vi "Decompose Map - Variant Value - Decomposes Successfully.vi"() -> ()   [LabVIEW 2019]
uses:
  <vilib>/addons/_JKI Toolkits/Caraya/classes/Assert/Assert Equal Value_Variant.vi
  Composition/Composition.lvlib
  <vilib>/addons/_JKI Toolkits/Caraya/classes/Test/Test.lvclass
  <vilib>/addons/_JKI Toolkits/Caraya/classes/Assert/Assert.lvclass
panel:
  out "error out":errorcluster
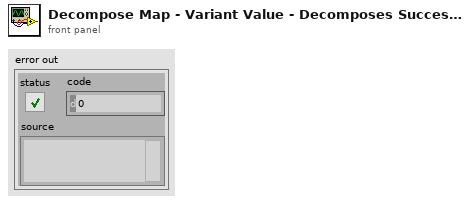
[diagram p1: front panel]
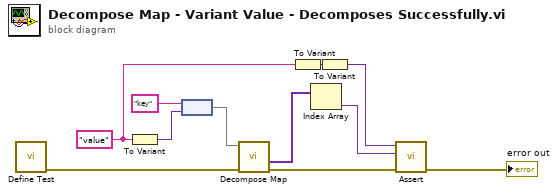
[diagram p0: block diagram]
diagram:
  w8 = "value" ("key")
  n1 = call <vilib>:"Define Test.vi"() -> ("error out"=w6:errorcluster)  [unwired: 10 in, 1 out]
  n2 = To Variant(anything=w8) -> (Variant=w5:variant)
  n3 = node("key" ("key"), w5) -> (w4:map{string, variant})
  n4 = call "Decompose Map.vi"("error in (no error)"=w6, "Variant Map"=w4) -> ("error out"=w10:errorcluster, "Values"=w3:variant[])  [unwired: 6 in, 2 out]
  n5 = To Variant(anything=w8) -> (Variant=w2:variant)
  n6 = Index Array(array=w3) -> (element=w9:variant)  [unwired: 1 in]
  n7 = To Variant(anything=w2) -> (Variant=w1:variant)
  n8 = call-poly <vilib>:"Assert.vi"("error in (no error)"=w10, "Y"=w9, "X"=w1) -> ("error out"=→"error out":errorcluster)  [unwired: 7 in, 1 out]
